vi "Plot GPS Logfile (Keith Koch's conflicted copy 2013-05-10).vi"(1 "file path (dialog if empty)":path=path "C:/Users/ATV Project/Dropbox/Auto-Steering and Obstacle Avoidance System Project/Software/VI's/_Data/Log_Files(GPS)/GPS_LOG_5-6-2013_6-12 PM") -> (0 "Navigation Duration(s)":i32)   [LabVIEW 2011]
uses:
  <vilib>/Utility/file.llb/Read From Spreadsheet File (DBL).vi
  _GlobalVariables&Libraries/ATV Program Global Variables.vi
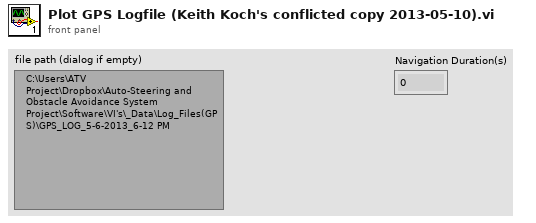
[diagram p1: front panel]
types:
  T1 = cluster{"Navigation Coordinates":cluster{"Latitude":dbl, "Longitude":dbl}[], "Coordinate Count":u32, "Drive Speed":string, "Steer Angle":dbl, "Steering":dbl, "Direction to next Coordinate":dbl, "Drive":dbl, "Navigation Path":string}
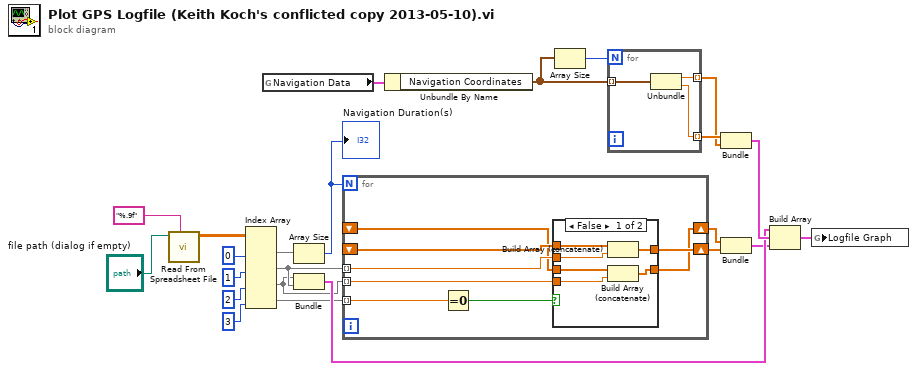
[diagram p0: block diagram]
diagram:
  n1 = call-poly <vilib>:"Read From Spreadsheet File.vi"("format (%.3f)"="%.9f", "file path (dialog if empty)"="file path (dialog if empty)") -> ("all rows"=w10:dbl[][])  [unwired: 5 in, 4 out]
  n2 = Index Array(array=w10, index (col) #1=0 ("disabled index (col)"), index (col) #2=1 ("index (col)"), index (col) #3=2 ("index (col)"), index (col) #4=3 ("index (col)")) -> (element #1=w9:dbl[], element #2=w5:dbl[], element #3=w4:dbl[], element #4=w6:dbl[])  [unwired: 4 in]
  n3 = global read "ATV Program Global Variables.vi" "Navigation Data"() -> (w22:T1)
  n4 = Array Size(array=w9) -> (size(s)=w7:i32)
  "Navigation Duration(s)" <- w7
  n5 = Bundle("all rows"=w4, "all rows"=w5) -> (w12:cluster{"all rows":dbl[], "all rows":dbl[]})  [unwired: 1 in]
  n6 = for {
    N: w7 -> [_]
    tunnel: w6 -> [w31] mode=indexing
    tunnel: w5 -> [w26] mode=indexing
    tunnel: w4 -> [w27] mode=indexing
    shift-right: [w29] -> w1
    shift-left: _ -> [w28]
    shift-right: [w25] -> w2
    shift-left: _ -> [w24]
    n7 = Equal To 0?(x=w31) -> (x = 0?=w30:bool)
    n8 = case shown="False" w30 {
      tunnel: [w35 w39] -> w29
      tunnel: w28 -> [w32 w39]
      tunnel: w27 -> [w36 _]
      tunnel: w26 -> [w37 _]
      tunnel: [w34 w38] -> w25
      tunnel: w24 -> [w33 w38]
      frame False {
        n9 = Build Array (concatenate)(w32, w37) -> (w35:dbl[])
        n10 = Build Array (concatenate)(w33, w36) -> (w34:dbl[])
      }
      frame True {
      }
    }
  }
  n11 = Unbundle By Name(w22) -> ("Navigation Coordinates"=w20:cluster{"Latitude":dbl, "Longitude":dbl}[])
  n12 = Array Size(array=w20) -> (size(s)=w21:i32)
  n13 = for {
    N: w21 -> [_]
    tunnel: w20 -> [w42] mode=indexing
    tunnel: [w41] -> w18 mode=indexing
    tunnel: [w40] -> w19 mode=indexing
    n14 = Unbundle(w42) -> ("Latitude"=w41:dbl, "Longitude"=w40:dbl)
  }
  n15 = Bundle(w19, w18) -> (w17:cluster{dbl[], dbl[]})  [unwired: 1 in]
  n16 = Bundle(w2, w1) -> (w3:cluster{dbl[], dbl[]})  [unwired: 1 in]
  n17 = Build Array(w12, w17, w3) -> (w11:cluster{"all rows":dbl[], "all rows":dbl[]}[])
  n18 = global write "ATV Program Global Variables.vi" "Logfile Graph"(w11) -> ()
